vi "Inline VI Contents.vi"(8 "error in (no error)":errorcluster, 11 "SubVI in":refnum<vi>) -> (0 "error out":errorcluster)   [LabVIEW 2018]
doc: "Places the newly created (temp) subVI which wraps the assert vi inline."
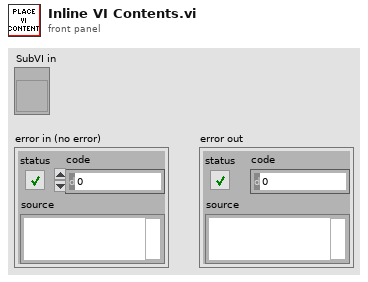
[diagram p1: front panel]
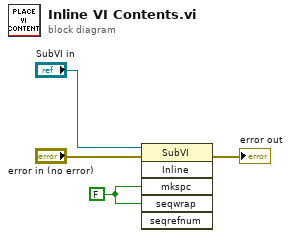
[diagram p0: block diagram]
diagram:
  w4 = FALSE ("Make Space in Block Diagram")
  n1 = invoke class="SubVI" method="Inline"(reference="SubVI in", error in="error in (no error)", "mkspc"=w4, "seqwrap"=w4) -> (error out=→"error out":errorcluster)  [unwired: 2 in, 5 out]
